vi "Do.vi"(8 "error in (no error)":errorcluster, 9 "Events":refnum<class "Events.lvclass">, 10 "Message Loop Data in":T1, 11 "IInternalRequest in":refnum<class "IRegisteredHandler.lvclass">) -> (0 "error out":errorcluster, 2 "Message Loop Data out":T1, 3 "IInternalRequest out":refnum<class "IRegisteredHandler.lvclass">)   [LabVIEW 2020, in "wamplv.lvlib" / "IRegisteredHandler.lvclass"]
uses:
  IRegisteredHandler.lvclass
  Message loop classes/ErrorOrSuccess/ErrorOrSuccess.lvclass
  WAMP Client/Private/TypeDef/Endpoint Data.ctl
  wamplv.lvlib
  Register/IRegister/IRegister.lvclass
  WAMP Client/Private/TypeDef/Publish Requests Map.ctl
  Call/ICallRequest/ICallRequest.lvclass
  WAMP Client/Private/TypeDef/CALL Request Map.ctl
  WAMP Client/Private/TypeDef/SUBSCRIBE Requests Map.ctl
  WAMP Client/Private/TypeDef/Subscriptions Map.ctl
  WAMP Client/Private/TypeDef/Unsubscribe Requests Map.ctl
  WAMP Client/Private/TypeDef/Unregister requests map.ctl
  WAMP Client/Private/TypeDef/Message Loop Data.ctl
  Events/EventsParent/Events.lvclass
  Subscribe/ISubscribe/ISubscribe.lvclass
  Publish/IPublish/IPublish.lvclass
  Message loop classes/Subscription details/SubscriptionDetailsParent/SubscriptionDetailsParent.lvclass
  Unsubscribe/IUnsubscribe/IUnsubscribe.lvclass
  Unregister/IUnregister/IUnregister.lvclass
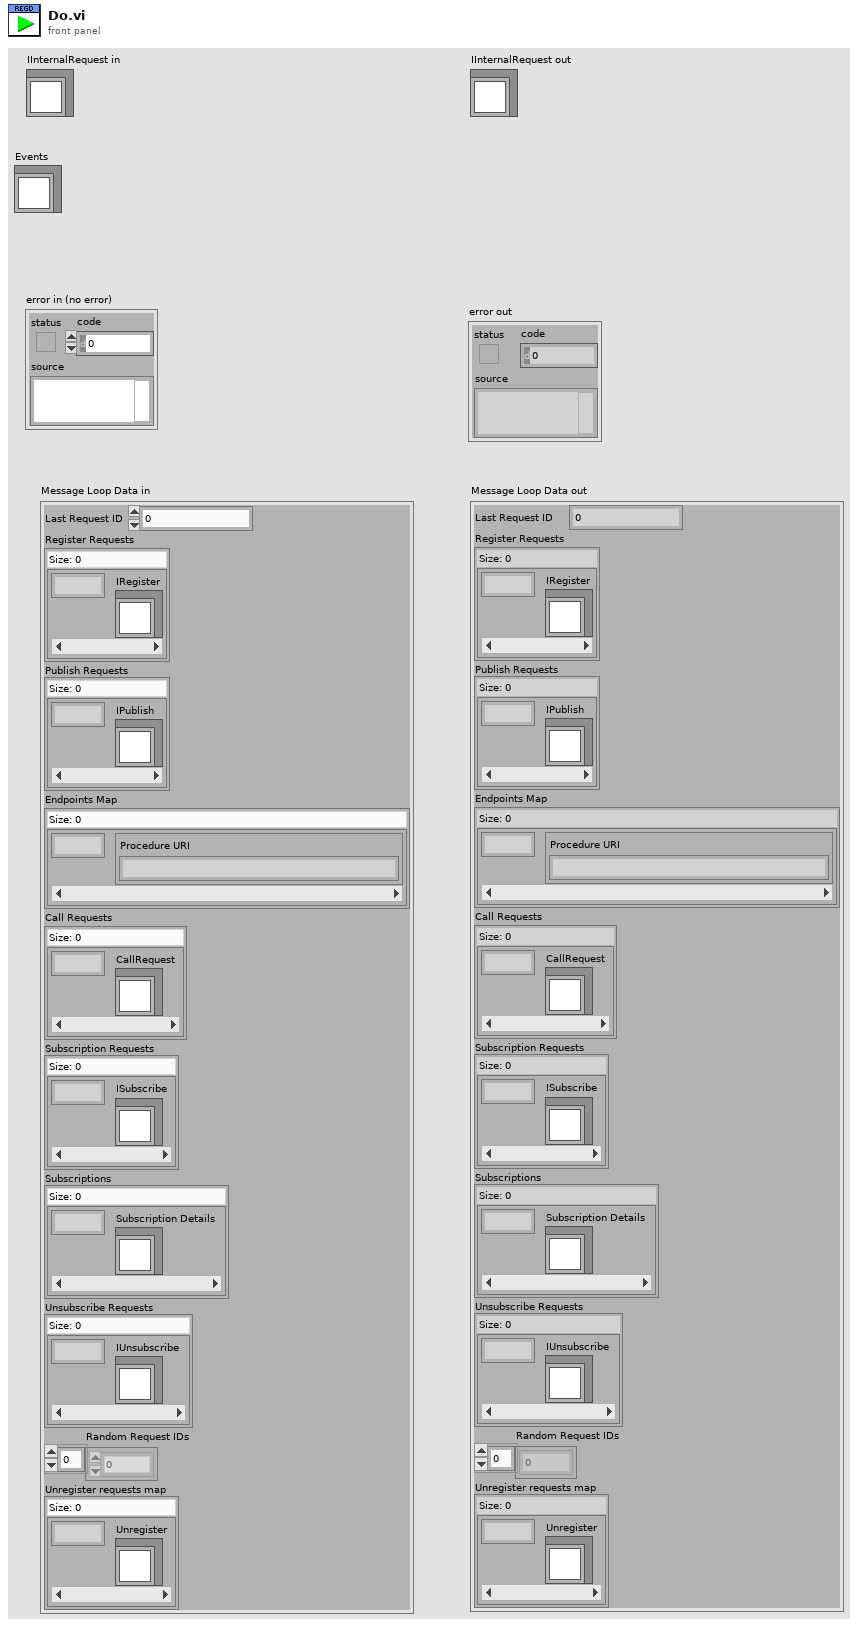
[diagram p1: front panel]
types:
  T1 = typedef "wamplv.lvlib/Message Loop Data.ctl" = cluster{"Last Request ID":u64, "Register Requests":map{u64, refnum<class "IRegister.lvclass">}, "Publish Requests":T2, "Endpoints Map":map{u64, T3}, "Call Requests":T4, "Subscription Requests":T5, "Subscriptions":T6, "Unsubscribe Requests":T7, "Random Request IDs":u64[], "Unregister requests map":T8}
  T2 = typedef "wamplv.lvlib/Publish Requests Map.ctl" = map{u64, refnum<class "IPublish.lvclass">}
  T3 = typedef "wamplv.lvlib/Endpoint Data.ctl" = cluster{"Procedure URI":string}
  T4 = typedef "wamplv.lvlib/CALL Request Map.ctl" = map{u64, refnum<class "ICallRequest.lvclass">}
  T5 = typedef "wamplv.lvlib/SUBSCRIBE Requests Map.ctl" = map{u64, refnum<class "ISubscribe.lvclass">}
  T6 = typedef "wamplv.lvlib/Subscriptions Map.ctl" = map{u64, refnum<class "SubscriptionDetailsParent.lvclass">}
  T7 = typedef "wamplv.lvlib/Unsubscribe Requests Map.ctl" = map{u64, refnum<class "IUnsubscribe.lvclass">}
  T8 = typedef "wamplv.lvlib/Unregister requests map.ctl" = map{u64, refnum<class "IUnregister.lvclass">}
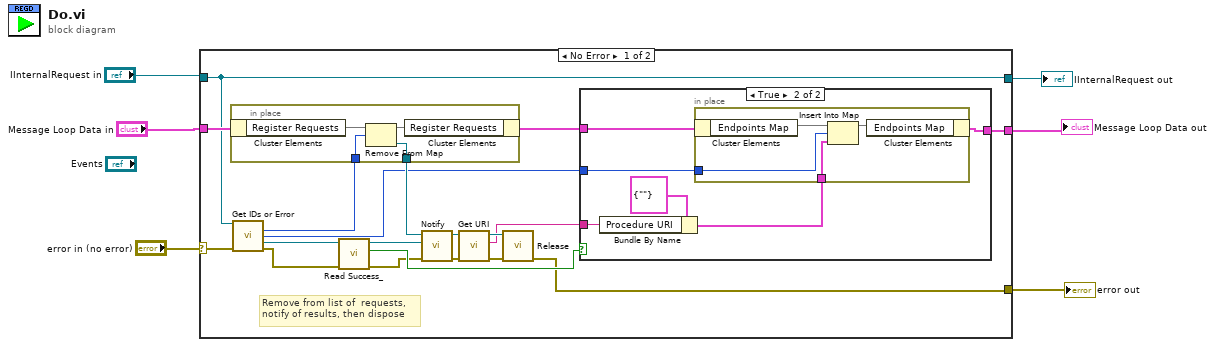
[diagram p0: block diagram]
diagram:
  n1 = case shown="No Error" "error in (no error)" {
    selector: "error in (no error)" -> [w20 w40]
    tunnel: "Message Loop Data in" -> [w24 w41]
    tunnel: [w7 w40] -> w1
    tunnel: [w21 w41] -> w2
    tunnel: "IInternalRequest in" -> [w19 w42]
    tunnel: [w19 w42] -> w3
    frame No Error {
      # "Remove from list of  requests,\nnotify of results, then dispose"
      n2 = call-dynamic "Get IDs or Error.vi"("IRegisteredHandler in"=w19, "error in (no error)"=w20) -> ("Request ID"=w18:u64, "Registration ID"=w9:u64, "ErrorOrSuccess"=w13:refnum<class "ErrorOrSuccess.lvclass">, "error out"=w17:errorcluster)  [unwired: 9 in, 1 out]
      n3 = in-place "In Place Element Structure" {
        in-place-border: w18 -> [w37]
        in-place-border: [w36] -> w16
        n4 = in-place-cluster #1(w24) -> ("Register Requests"=w39:map{u64, refnum<class "IRegister.lvclass">})
        n5 = Remove From Map(10:w37, 11:w39) -> (1:w36:refnum<class "IRegister.lvclass">, 3:w38:map{u64, refnum<class "IRegister.lvclass">})  [unwired: 1 out]
        n6 = in-place-cluster #1("Register Requests"=w38) -> (w23:T1)
      }
      n7 = call "Read Success_.vi"("error in (no error)"=w17, "ErrorOrSuccess in"=w13) -> ("error out"=w15:errorcluster, "Success?"=w22:bool, "ErrorOrSuccess out"=w12:refnum<class "ErrorOrSuccess.lvclass">)  [unwired: 7 in]
      n8 = call-dynamic "Notify.vi"("error in (no error)"=w15, "ErrorOrSuccess"=w12, "IRegister in"=w16) -> ("error out"=w14:errorcluster, "IRegister out"=w11:refnum<class "IRegister.lvclass">)  [unwired: 7 in]
      n9 = call-dynamic "Get URI.vi"("IRegister in"=w11) -> ("URI"=w8:string, "IRegister out"=w10:refnum<class "IRegister.lvclass">)  [unwired: 9 in]
      n10 = call-dynamic "Release.vi"("error in (no error)"=w14, "IContainersNotiferOrEvents in"=w10) -> ("error out"=w7:errorcluster)  [unwired: 9 in]
      n11 = case shown="True" w22 {
        tunnel: w23 -> [w25 w30]
        tunnel: [w25 w31] -> w21
        tunnel: w9 -> [_ w29]
        tunnel: w8 -> [_ w26]
        frame False {
        }
        frame True {
          n12 = Bundle By Name(cluster=T3 {"Procedure URI"=""} ("value"), "Procedure URI"=w26) -> (w27:T3)
          n13 = in-place {
            in-place-border: w29 -> [w33]
            in-place-border: w27 -> [w32]
            n14 = in-place-cluster #2(w30) -> ("Endpoints Map"=w35:map{u64, T3})
            n15 = Insert Into Map(map in=w35, key=w33, value=w32) -> (map out=w34:map{u64, T3})  [unwired: 2 out]
            n16 = in-place-cluster #2("Endpoints Map"=w34) -> (w31:T1)
          }
        }
      }
    }
    frame Error {
    }
  }
  "error out" <- w1
  "IInternalRequest out" <- w3
  "Message Loop Data out" <- w2
